vi "Stop Core.vi"(10 "final error code":i32, 11 "VG-VNA_GUI in":refnum<class "VG-VNA_GUI.lvclass">) -> (3 "VG-VNA_GUI out":refnum<class "VG-VNA_GUI.lvclass">)   [LabVIEW 2020, in "VG-VNA_GUI.lvlib" / "VG-VNA_GUI.lvclass"]
doc: "(<B>Filename</B>: Actor Framework.lvlib:Actor.lvclass:Stop Core.vi)\n\nDefines what the actor does before it stops. Use the <B>final error code</B> input to determine whether the actor shut down in response to an error.\n\nBy default, this method passes the Stop message along to all auto-stop nested actors. A descendant class may override this method to define additional behavior, such as shutting down any processes the actor initiated in its override of the Actor Core method."
uses:
  VG-VNA_GUI.lvclass
  <vilib>/ActorFramework/Actor/Actor.lvclass
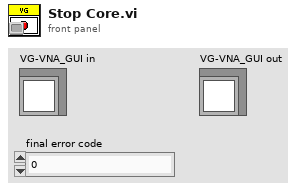
[diagram p1: front panel]
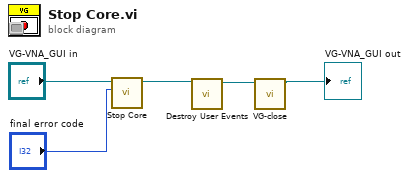
[diagram p0: block diagram]
diagram:
  n1 = call-parent "Stop Core.vi"("final error code"="final error code", "Actor in"="VG-VNA_GUI in") -> ("Actor out"=w2:refnum<class "VG-VNA_GUI.lvclass">)  [unwired: 9 in]
  n2 = call "Destroy User Events.vi"("VG-VNA_GUI in"=w2) -> ("VG-VNA_GUI out"=w1:refnum<class "VG-VNA_GUI.lvclass">)  [unwired: 10 in]
  n3 = call "VG-close.vi"("VG-VNA_GUI in"=w1) -> ("VG-VNA_GUI out"=→"VG-VNA_GUI out":refnum<class "VG-VNA_GUI.lvclass">)  [unwired: 10 in]
